vi "wsGetSingleState.vi"(8 "error in (no error)":errorcluster, 11 "JSON String":string) -> (0 "error out":errorcluster, 3 "State":T1)   [LabVIEW 2018, in "HASS-LV-WS_integration.lvlib"]
uses:
  HASS-LV-WS_integration.lvlib
  <vilib>/addons/_JKI.lib/Serialization/JSON/JKI JSON Serialization.lvlib
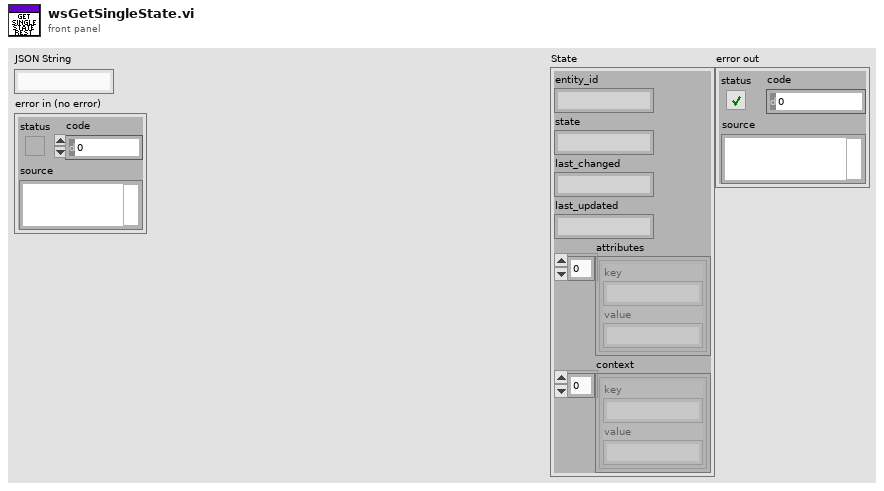
[diagram p1: front panel]
types:
  T1 = cluster{"entity_id":string, "state":string, "last_changed":string, "last_updated":string, "attributes":cluster{"key":string, "value":string}[], "context":cluster{"key":string, "value":string}[]}
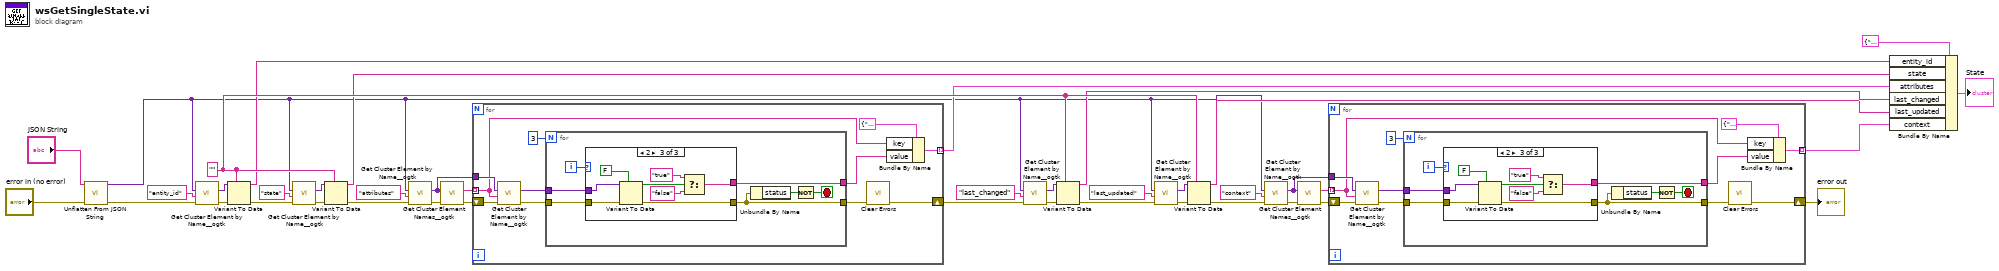
[diagram p0: block diagram]
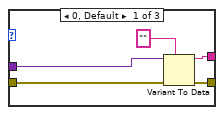
[diagram p2: hidden frame]
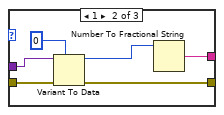
[diagram p3: hidden frame]
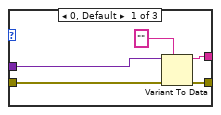
[diagram p4: hidden frame]
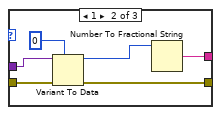
[diagram p5: hidden frame]
diagram:
  w22 = ""
  n1 = call <vilib>:"Unflatten From JSON String.vi"("error in (no error)"="error in (no error)", "JSON String"="JSON String") -> ("error out"=w2:errorcluster, "Variant"=w1:variant)  [unwired: 8 in]
  n2 = call <userlib>:"Get Cluster Element by Name__ogtk.vi"("error in (no error)"=w2, "Element Name"="entity_id", "Cluster"=w1) -> ("error out"=w34:errorcluster, "VElement"=w26:variant)  [unwired: 6 in, 1 out]
  n3 = Variant To Data(error in=w34, type=w22, Variant=w26) -> (data=w20:string, error out=w33:errorcluster)
  n4 = call <userlib>:"Get Cluster Element by Name__ogtk.vi"("error in (no error)"=w33, "Element Name"="state", "Cluster"=w1) -> ("error out"=w32:errorcluster, "VElement"=w25:variant)  [unwired: 6 in, 1 out]
  n5 = Variant To Data(error in=w32, type=w22, Variant=w25) -> (data=w19:string, error out=w31:errorcluster)
  n6 = call <userlib>:"Get Cluster Element by Name__ogtk.vi"("error in (no error)"=w31, "Element Name"="attributes", "Cluster"=w1) -> ("error out"=w14:errorcluster, "VElement"=w16:variant)  [unwired: 6 in, 1 out]
  n7 = call <userlib>:"Get Cluster Element Names__ogtk.vi"("error in (no error)"=w14, "Cluster"=w16) -> ("error out"=w13:errorcluster, "Element Names"=w15:string[])  [unwired: 8 in]
  n8 = for {
    tunnel: w16 -> [w52]
    tunnel: w15 -> [w47] mode=indexing
    shift-right: [w42] -> w12
    shift-left: w13 -> [w49]
    tunnel: [w46] -> w11 mode=indexing
    n9 = call <userlib>:"Get Cluster Element by Name__ogtk.vi"("error in (no error)"=w49, "Element Name"=w47, "Cluster"=w52) -> ("error out"=w51:errorcluster, "VElement"=w44:variant)  [unwired: 6 in, 1 out]
    n10 = for {
      N: 3 -> [_]
      tunnel: [w58] -> w45
      tunnel: w44 -> [w57]
      tunnel: w51 -> [w59]
      tunnel: [w55] -> w50
      i -> [w56]
      stop <- w53 stop-if-true
      n11 = case shown="2" w56 {
        tunnel: w59 -> [w60 w70 w78]
        tunnel: [w61 w67 w76] -> w55
        tunnel: [w62 w65 w72] -> w58
        tunnel: w57 -> [w63 w69 w77]
        frame 0, Default {
          n12 = Variant To Data(error in=w60, type="", Variant=w63) -> (data=w62:string, error out=w61:errorcluster)
        }
        frame 1 {
          n13 = Variant To Data(error in=w70, type=0, Variant=w69) -> (data=w66:i32, error out=w67:errorcluster)
          n14 = Number To Fractional String(number=w66) -> (F-format string=w65:string)  [unwired: 3 in]
        }
        frame 2 {
          n15 = Variant To Data(error in=w78, type=FALSE, Variant=w77) -> (data=w74:bool, error out=w76:errorcluster)
          n16 = Select(t="true", s=w74, f="false") -> (s? t:f=w72:string)
        }
      }
      n17 = Unbundle By Name(w55) -> ("status"=w54:bool)
      n18 = Not(x=w54) -> (.not. x?=w53:bool)
    }
    n19 = call <vilib>:"Clear Errors.vi"("error in (no error)"=w50) -> ("error out"=w42:errorcluster)  [unwired: 5 in, 1 out]
    n20 = Bundle By Name(cluster=cluster{"key":string, "value":string} {"key"="", "value"=""}, "key"=w47, "value"=w45) -> (w46:cluster{"key":string, "value":string})
  }
  n21 = call <userlib>:"Get Cluster Element by Name__ogtk.vi"("error in (no error)"=w12, "Element Name"="last_changed", "Cluster"=w1) -> ("error out"=w30:errorcluster, "VElement"=w24:variant)  [unwired: 6 in, 1 out]
  n22 = Variant To Data(error in=w30, type=w22, Variant=w24) -> (data=w18:string, error out=w29:errorcluster)
  n23 = call <userlib>:"Get Cluster Element by Name__ogtk.vi"("error in (no error)"=w29, "Element Name"="last_updated", "Cluster"=w1) -> ("error out"=w28:errorcluster, "VElement"=w23:variant)  [unwired: 6 in, 1 out]
  n24 = Variant To Data(error in=w28, type=w22, Variant=w23) -> (data=w17:string, error out=w27:errorcluster)
  n25 = call <userlib>:"Get Cluster Element by Name__ogtk.vi"("error in (no error)"=w27, "Element Name"="context", "Cluster"=w1) -> ("error out"=w10:errorcluster, "VElement"=w7:variant)  [unwired: 6 in, 1 out]
  n26 = call <userlib>:"Get Cluster Element Names__ogtk.vi"("error in (no error)"=w10, "Cluster"=w7) -> ("error out"=w9:errorcluster, "Element Names"=w8:string[])  [unwired: 8 in]
  n27 = for {
    tunnel: w7 -> [w89]
    tunnel: w8 -> [w86] mode=indexing
    shift-right: [w80] -> w4
    shift-left: w9 -> [w88]
    tunnel: [w85] -> w6 mode=indexing
    n28 = call <userlib>:"Get Cluster Element by Name__ogtk.vi"("error in (no error)"=w88, "Element Name"=w86, "Cluster"=w89) -> ("error out"=w84:errorcluster, "VElement"=w83:variant)  [unwired: 6 in, 1 out]
    n29 = for {
      N: 3 -> [_]
      tunnel: [w95] -> w81
      tunnel: w83 -> [w94]
      tunnel: w84 -> [w96]
      tunnel: [w92] -> w82
      i -> [w93]
      stop <- w90 stop-if-true
      n30 = case shown="2" w93 {
        tunnel: w96 -> [w97 w107 w115]
        tunnel: [w98 w104 w113] -> w92
        tunnel: [w99 w102 w109] -> w95
        tunnel: w94 -> [w100 w106 w114]
        frame 0, Default {
          n31 = Variant To Data(error in=w97, type="", Variant=w100) -> (data=w99:string, error out=w98:errorcluster)
        }
        frame 1 {
          n32 = Variant To Data(error in=w107, type=0, Variant=w106) -> (data=w103:i32, error out=w104:errorcluster)
          n33 = Number To Fractional String(number=w103) -> (F-format string=w102:string)  [unwired: 3 in]
        }
        frame 2 {
          n34 = Variant To Data(error in=w115, type=FALSE, Variant=w114) -> (data=w111:bool, error out=w113:errorcluster)
          n35 = Select(t="true", s=w111, f="false") -> (s? t:f=w109:string)
        }
      }
      n36 = Unbundle By Name(w92) -> ("status"=w91:bool)
      n37 = Not(x=w91) -> (.not. x?=w90:bool)
    }
    n38 = call <vilib>:"Clear Errors.vi"("error in (no error)"=w82) -> ("error out"=w80:errorcluster)  [unwired: 5 in, 1 out]
    n39 = Bundle By Name(cluster=cluster{"key":string, "value":string} {"key"="", "value"=""}, "key"=w86, "value"=w81) -> (w85:cluster{"key":string, "value":string})
  }
  "error out" <- w4
  n40 = Bundle By Name(cluster=T1 {"entity_id"="", "state"="", "last_changed"="", "last_updated"="", "attributes"=[], "context"=[]}, "entity_id"=w20, "state"=w19, "attributes"=w11, "last_changed"=w18, "last_updated"=w17, "context"=w6) -> (→"State":T1)
